vi "decorrelaton_curve_Ascans.vi"(6 "Num averages":i32=10, 7 "Num Shifts":i32, 9 "ROI Height":dbl, 10 "ROI Depth":dbl, 11 "Image":T1) -> (2 "spacing":dbl, 3 "correlation":dbl)   [LabVIEW 2016]
uses:
  <vilib>/vision/Image Controls.llb/IMAQ Image.ctl
  <vilib>/Analysis/baseanly.llb/Mean (DBL).vi
  <vilib>/vision/NI_Vision_Development_Module.lvlib
  <vilib>/Analysis/NI_AALBase.lvlib
panel:
  out "Image 2":T1(plugin-control)
  out "Waveform Chart":dbl[](graph)
  out "peak column":i32
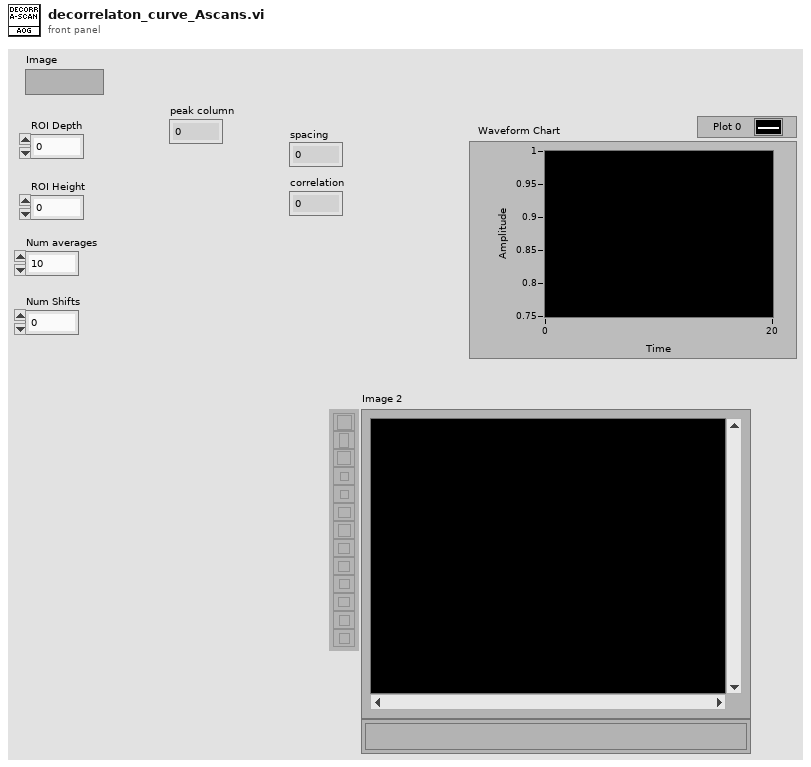
[diagram p1: front panel]
types:
  T1 = typedef "IMAQ Image.ctl" = refnum<image>
  T2 = typedef "Image Type" = u32
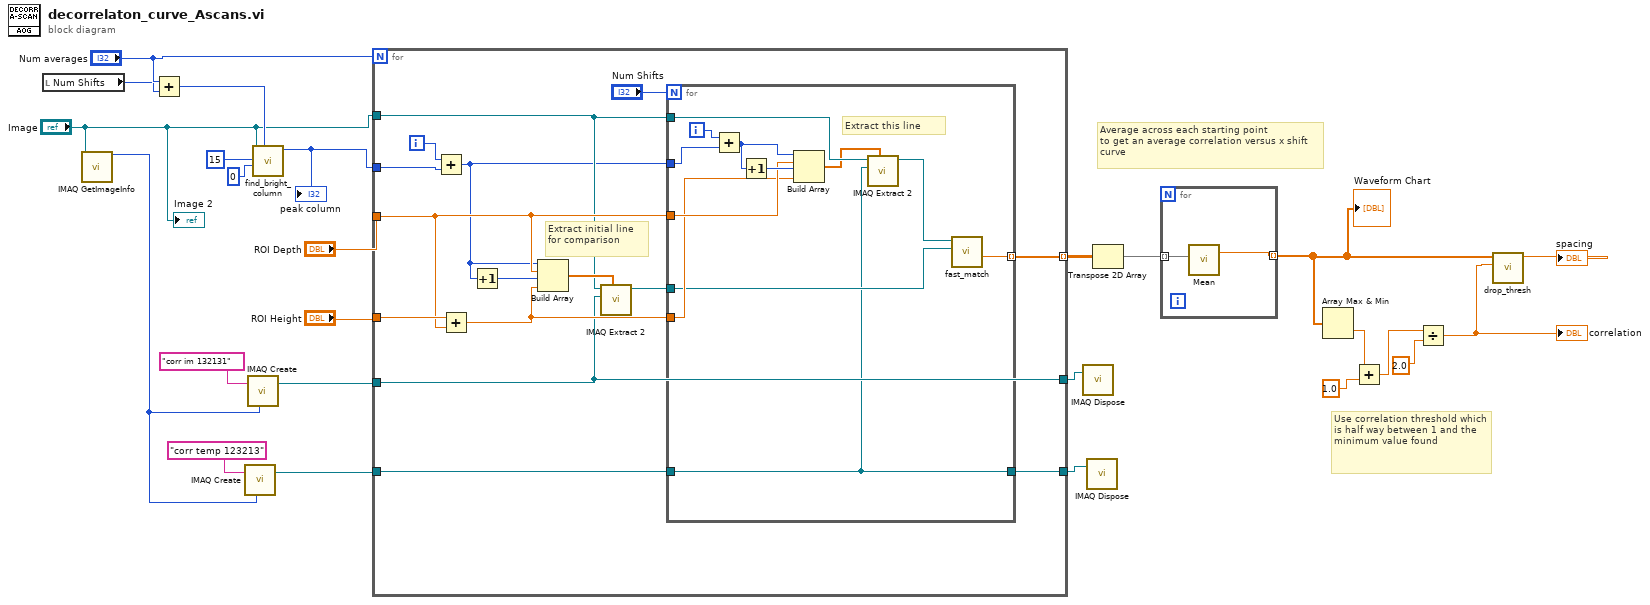
[diagram p0: block diagram]
diagram:
  # "Average across each starting point\nto get an average correlation versus x shift\ncurve"
  # "Use correlation threshold which is half way between 1 and the minimum value found"
  n1 = local read "Num Shifts"() -> (w9:i32)
  n2 = call "IMAQ GetImageInfo"("Image"="Image") -> ("Image Type"=w13:T2)  [unwired: 3 in, 7 out]
  n3 = Add(x="Num averages", y=w9) -> (x+y=w8:i32)
  n4 = call "IMAQ Create"("Image Name"="corr temp 123213", "Image Type"=w13) -> ("New Image"=w20:T1)  [unwired: 3 in, 1 out]
  n5 = call "IMAQ Create"("Image Name"="corr im 132131", "Image Type"=w13) -> ("New Image"=w21:T1)  [unwired: 3 in, 1 out]
  n6 = call "find_bright_column.vi"("Right border"=w8, "Left border"=0, "filter size"=15, "Image"="Image") -> ("peak column"=w5:i32)  [unwired: 7 in]
  "peak column" <- w5
  n7 = for {
    N: "Num averages" -> [_]
    tunnel: "ROI Height" -> [w40]
    tunnel: w5 -> [w30]
    tunnel: "ROI Depth" -> [w37]
    tunnel: "Image" -> [w35]
    tunnel: w21 -> [w27]
    tunnel: w20 -> [w34]
    tunnel: [w33] -> w15 mode=indexing
    tunnel: [w27] -> w11
    tunnel: [w26] -> w12
    i -> [w29]
    # "Extract initial line for comparison"
    n8 = Add(x=w29, y=w30) -> (x+y=w31:i32)
    n9 = Add(x=w40, y=w37) -> (x+y=w36:dbl)
    n10 = Increment(x=w31) -> (x+1=w39:i32)
    n11 = Build Array(w31, w37, w39, w36) -> (w38:dbl[])
    n12 = call "IMAQ Extract 2"("Optional Rectangle"=w38, "Image Dst"=w27, "Image Src"=w35) -> ("Image Dst Out"=w32:T1)  [unwired: 7 in, 1 out]
    n13 = for {
      N: "Num Shifts" -> [_]
      tunnel: w35 -> [w46]
      tunnel: w31 -> [w51]
      tunnel: w37 -> [w48]
      tunnel: w36 -> [w47]
      tunnel: w34 -> [w41]
      tunnel: w32 -> [w43]
      tunnel: [w42] -> w33 mode=indexing
      tunnel: [w41] -> w26
      i -> [w52]
      # "Extract this line"
      n14 = Add(x=w52, y=w51) -> (x+y=w49:i32)
      n15 = Increment(x=w49) -> (x+1=w50:i32)
      n16 = Build Array(w49, w48, w50, w47) -> (w45:dbl[])
      n17 = call "IMAQ Extract 2"("Optional Rectangle"=w45, "Image Dst"=w41, "Image Src"=w46) -> ("Image Dst Out"=w44:T1)  [unwired: 7 in, 1 out]
      n18 = call "fast_match.vi"("Template"=w43, "Image"=w44) -> ("score"=w42:dbl)  [unwired: 6 in, 3 out]
    }
  }
  n19 = call "IMAQ Dispose"("Image"=w11) -> ()  [unwired: 5 in, 1 out]
  n20 = call "IMAQ Dispose"("Image"=w12) -> ()  [unwired: 5 in, 1 out]
  n21 = Transpose 2D Array(2D array=w15) -> (transposed array=w14:dbl[][])
  n22 = for {
    tunnel: w14 -> [w54] mode=indexing
    tunnel: [w53] -> w1 mode=indexing
    n23 = call-poly <vilib>:"Mean.vi"("X"=w54) -> ("mean"=w53:dbl)  [unwired: 1 out]
  }
  "Waveform Chart" <- w1
  n24 = Array Max & Min(array=w1) -> (min value=w17:dbl)  [unwired: 3 out]
  n25 = Add(x=w17, y=1.0) -> (x+y=w16:dbl)
  n26 = Divide(x=w16, y=2.0) -> (x/y=w3:dbl)
  "correlation" <- w3
  n27 = call "drop_thresh.vi"("threshold"=w3, "curve"=w1) -> ("position"=→"spacing":dbl)  [unwired: 9 in]
  "Image 2" <- "Image"
